vi "Calc_Parallel_Resitance.vi"(11 "Resitance_Per Site":dbl[](array[numeric])) -> (3 "Parralel_Resistance":dbl[](array[numeric]))   [LabVIEW 2013]
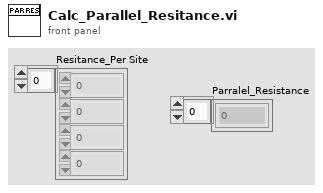
[diagram p1: front panel]
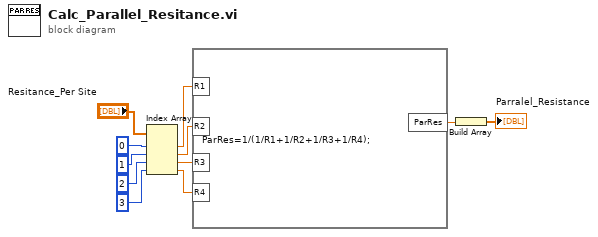
[diagram p0: block diagram]
diagram:
  n1 = Index Array(array="Resitance_Per Site", index #1=0 ("index"), index #2=1 ("index"), index #3=2 ("index"), index #4=3 ("index")) -> (element #1=w6:dbl, element #2=w5:dbl, element #3=w4:dbl, element #4=w3:dbl)
  n2 = formula code="ParRes=1/(1/R1+1/R2+1/R3+1/R4);"("R1"=w6, "R2"=w5, "R3"=w4, "R4"=w3) -> ("ParRes"=w2:dbl)
  n3 = Build Array(w2) -> (→"Parralel_Resistance":dbl[])
